vi "Get Relay Names.vi"(8 "error in (no error)":errorcluster, 11 "SLSC Switch in":refnum<class "SLSC Switch.lvclass">) -> (0 "error out":errorcluster, 2 "Relay Names":string[](array[string]), 3 "SLSC Switch out":refnum<class "SLSC Switch.lvclass">)   [LabVIEW 2015, in "SLSC Switch.lvclass"]
doc: "Retrurns a list of all relays available on the card."
uses:
  SLSC Switch.lvclass
  SLSC Switch.lvclass/SLSC Switch.ctl
  Relay Interface/RelayInterface.lvclass
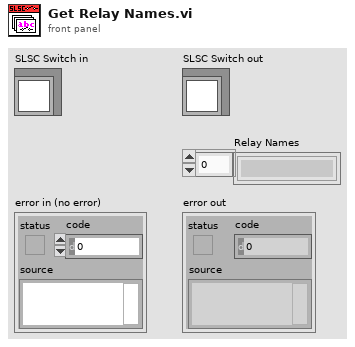
[diagram p1: front panel]
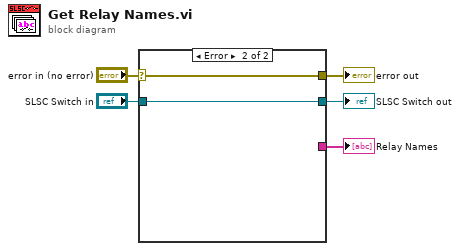
[diagram p0: block diagram]
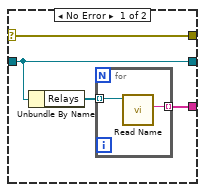
[diagram p2: hidden frame]
diagram:
  n1 = case shown="Error" "error in (no error)" {
    selector: "error in (no error)" -> [w9 w13]
    tunnel: [w9 w13] -> w4
    tunnel: [w8 _] -> w3
    tunnel: "SLSC Switch in" -> [w7 w12]
    tunnel: [w7 w12] -> w1
    frame No Error {
      n2 = Unbundle By Name(w7) -> ("Relays"=w6:refnum<class "RelayInterface.lvclass">[])
      n3 = for {
        tunnel: w6 -> [w11] mode=indexing
        tunnel: [w10] -> w8 mode=indexing
        n4 = call-dynamic "Read Name.vi"("RelayInterface in"=w11) -> ("Name"=w10:string)  [unwired: 9 in, 1 out]
      }
    }
    frame Error {
    }
  }
  "error out" <- w4
  "Relay Names" <- w3
  "SLSC Switch out" <- w1
